vi "Ex5.vi"() -> ()   [LabVIEW 2019]
panel:
  in  "stop":bool
  in  "consigne":dbl(slide) scale=0.0..1100.0
  out "Tank":dbl(slide) scale=0.0..1100.0
  in  "Consigne Num":dbl min=0.0 max=1100.0 format="%#_6f"
  out "?":dbl
  in  "Débit":dbl(slide) scale=1.0..10.0
  # "[l/s]"
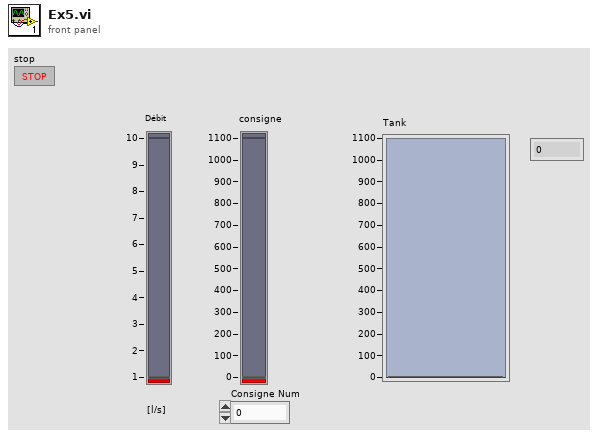
[diagram p1: front panel]
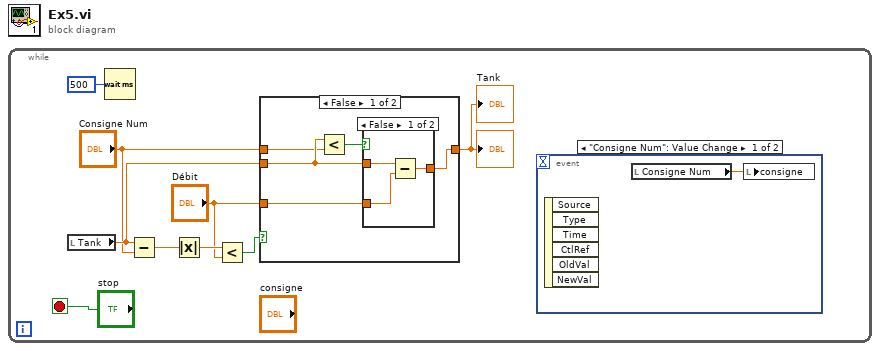
[diagram p0: block diagram]
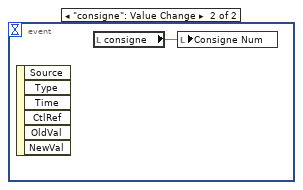
[diagram p2: hidden frame]
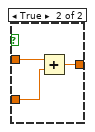
[diagram p3: hidden frame]
diagram:
  n1 = while {
    stop <- "stop" stop-if-true
    n2 = local read "Tank"() -> (w5:dbl)
    n3 = Wait (ms)(milliseconds to wait=500) -> ()  [unwired: 1 out]
    n4 = Subtract(x=w5, y="Consigne Num") -> (x-y=w8:dbl)
    n5 = Absolute Value(x=w8) -> (abs(x)=w7:dbl)
    n6 = Less?(x=w7, y="Débit") -> (x < y?=w6:bool)
    n7 = case shown="False" w6 {
      tunnel: [w14 w23] -> w3
      tunnel: "Consigne Num" -> [w12 w23]
      tunnel: w5 -> [w15 _]
      tunnel: "Débit" -> [w13 _]
      frame False {
        n8 = Less?(x=w15, y=w12) -> (x < y?=w16:bool)
        n9 = case shown="False" w16 {
          tunnel: w15 -> [w19 w22]
          tunnel: w13 -> [w18 w21]
          tunnel: [w17 w20] -> w14
          frame False {
            n10 = Subtract(x=w19, y=w18) -> (x-y=w17:dbl)
          }
          frame True {
            n11 = Add(x=w22, y=w21) -> (x+y=w20:dbl)
          }
        }
      }
      frame True {
      }
    }
    "Tank" <- w3
    "?" <- w3
    n12 = event shown="[0] \"Consigne Num\": Value Change" {
      selector: _ -> [_ _]
      dyn-events: _ -> [_ _]
      timeout: _ -> [_ _]
      event "Consigne Num": Value Change {
        n13 = event-data() -> ()  [unwired: 1 in, 6 out]
        n14 = local read "Consigne Num"() -> (w10:dbl)
        n15 = local write "consigne"(w10) -> ()
      }
      event "consigne": Value Change {
        n16 = event-data() -> ()  [unwired: 1 in, 6 out]
        n17 = local read "consigne"() -> (w11:dbl)
        n18 = local write "Consigne Num"(w11) -> ()
      }
    }
  }
